vi "Write Numeric Scalar to Source (Base16 I8).vi"(9 "offset":i32, 10 "value":i8, 11 "error in":errorcluster) -> (1 "new offset":i32, 3 "error out":errorcluster)   [LabVIEW 2017, in "Static Error Handling.lvlib"]
doc: "Converts <b>value</b> into an hexadecimal-formatted string, and writes the string to the <b>error in</b> source buffer at the specified <b>offset</b>."
uses:
  Static Error Handling.lvlib
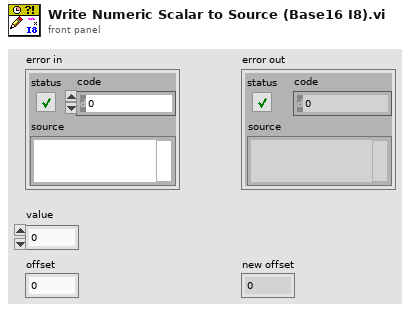
[diagram p1: front panel]
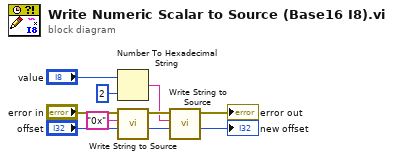
[diagram p0: block diagram]
diagram:
  n1 = Number To Hexadecimal String(1:i16 2 ("width (-)"), 2:"value") -> (0:w1:string)
  n2 = call "Write String to Source.vi"("offset"="offset", "string"="0x", "error in"="error in") -> ("new offset"=w2:i32, "error out"=w3:errorcluster)  [unwired: 7 in]
  n3 = call "Write String to Source.vi"("offset"=w2, "string"=w1, "error in"=w3) -> ("new offset"=→"new offset":i32, "error out"=→"error out":errorcluster)  [unwired: 7 in]
